vi "Get Start Up Time.vi"(11 "time":sgl) -> (2 "function return":u32, 3 "time out":sgl)   [LabVIEW 2018, in "AndorSDK.lvlib"]
doc: "EXPNETTYPE unsigned int WINAPI GetStartUpTime(float * time);"
uses:
  AndorSDK.lvlib
  ATMCD32D.dll
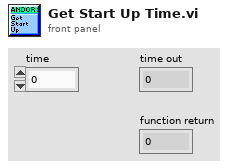
[diagram p1: front panel]
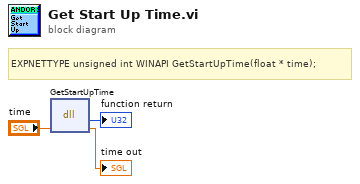
[diagram p0: block diagram]
diagram:
  # "EXPNETTYPE unsigned int WINAPI GetStartUpTime(float * time);"
  n1 = dll-call lib="PTH2babs E\nPersönliches02 - Arbeit03-HiwijobsLabviewCodelibANDOR\tAndor SDK\nATMCD32D.*" fn="GetStartUpTime"("time"="time") -> (→"function return":u32, "time"=→"time out":sgl)  [unwired: 3 in, 2 out]
